vi "RaspilArray (SubVI).vi"(11 "Array 3":dbl[][](array[numeric])) -> (1 "All GLUBIN":dbl[](array[numeric]), 2 "Array 2":dbl[][](array[numeric]), 3 "ZnachChastot":dbl[](array[numeric]), 4 "Array":dbl[](array[numeric]), 5 "Chastota":dbl[](array[numeric]))   [LabVIEW 2017]
uses:
  <vilib>/Analysis/NI_AALPro.lvlib
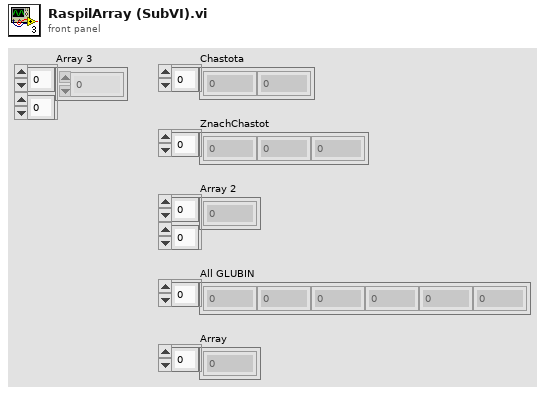
[diagram p1: front panel]
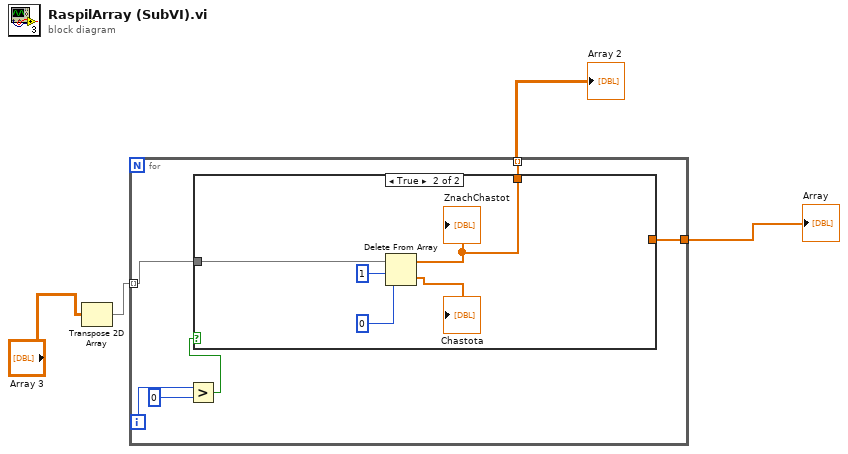
[diagram p0: block diagram]
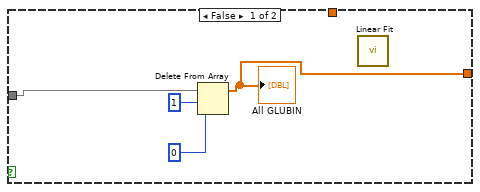
[diagram p2: hidden frame]
diagram:
  n1 = Transpose 2D Array(2D array="Array 3") -> (transposed array=w2:dbl[][])
  n2 = for {
    tunnel: w2 -> [w10] mode=indexing
    tunnel: [w6] -> w3 mode=indexing
    tunnel: [w5] -> w4
    i -> [w9]
    n3 = Greater?(x=w9, y=0) -> (0:w7:bool)
    n4 = case shown="True" w7 {
      tunnel: w10 -> [w12 w17]
      tunnel: [_ w15] -> w6
      tunnel: [w11 _] -> w5
      frame False {
        n5 = Delete From Array(array=w12, length=1, index=0) -> (array with subset deleted=w11:dbl[])  [unwired: 1 out]
        "All GLUBIN" <- w11
        n6 = call <vilib>:"Linear Fit.vi"() -> ()  [unwired: 11 in, 5 out]
      }
      frame True {
        n7 = Delete From Array(array=w17, length=1, index=0) -> (deleted portion=→"Chastota":dbl[], array with subset deleted=w15:dbl[])
        "ZnachChastot" <- w15
      }
    }
  }
  "Array" <- w4
  "Array 2" <- w3
